vi "re_LuaVIEW Run Task.vi"(0 "script file or name (no name)":path, 5 "custom search directory (none)":path, 7 "script string (\"\" == load from file)":string, 9 "manual? (false)":bool, 11 "error in (no error)":errorcluster) -> (4 "manual error":bool, 8 "identifier":string, 15 "error out":errorcluster)   [LabVIEW 2012]
doc: "Runs a new LuaVIEW task. This prepares a task and runs it. This VI returns when the task has progressed beyond its initialization. When the task fails while initializing, its error is returned."
uses:
  typedefs/t_LuaVIEW Task State Instantiator Methods.ctl
  typedefs/t_LuaVIEW Task State Methods.ctl
  typedefs/t_LuaVIEW Task Modes.ctl
  typedefs/t_LuaVIEW Task Signals.ctl
  typedefs/t_LuaVIEW Prepared Script Infos Methods.ctl
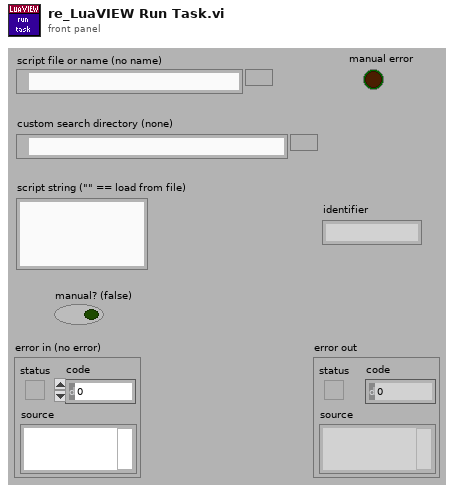
[diagram p1: front panel]
types:
  T1 = typedef "t_LuaVIEW Task State Instantiator Methods.ctl" = enum16{"instantiate", "isset", "retrieve"}
  T2 = typedef "t_LuaVIEW Task Modes.ctl" = enum16{"initializing", "running", "executing", "paused", "error", "swapping"}
  T3 = typedef "t_LuaVIEW Task State Methods.ctl" = enum16{"cleanup", "set initial", "set mode", "set active mode", "set error", "get task info", "get script info", "set signal", "clear signal", "test handled", "test delegated", "test signal", "handle signal", "delegate signal", "allow signal", "disallow signal", "disallow all", "signals?", "delegated signals?", "protection++", "protection--", "protection=0", "message", "next message", "pop message", "message available?", "force stop", "set swap preps", "apply swap preps"}
  T4 = typedef "t_LuaVIEW Task Signals.ctl" = enum32{"resume", "pause", "swap", "stop", "confirm"}
  T5 = typedef "t_LuaVIEW Prepared Script Infos Methods.ctl" = enum16{"isempty?", "empty", "set", "discard"}
  T6 = typedef "t_LuaVIEW Task State Pane.ctl" = refnum<vi>
  T7 = typedef "LuaVIEW Task Info.ctl" = cluster{"main script":string, "identifier":string, "class":string, "description":string, "mode":T2, "handler":string, "LuaVIEW reference":T8, "scripts":i32, "hide":bool, "active":bool, "error msg":string, "defer":bool, "launch":enum16{"asynchronous", "manual", "synchronous"}, "main path valid":bool, "start time":dbl, "swap time":dbl, "task VI":refnum<vi>, "prefsys":enum32{"invalid execution system", "user interface", "standard", "instrument i/o", "data acquisition", "other 1", "other 2", "same as caller"}, "priority":enum32{"invalid priority", "background priority", "normal priority", "above normal priority", "high priority", "time critical priority", "subroutine"}, "signal flags":u32, "allow mask":u32, "handle mask":u32, "disallow manual":bool}
  T8 = typedef "t_LuaVIEW Reference.ctl" = refnum<k1>
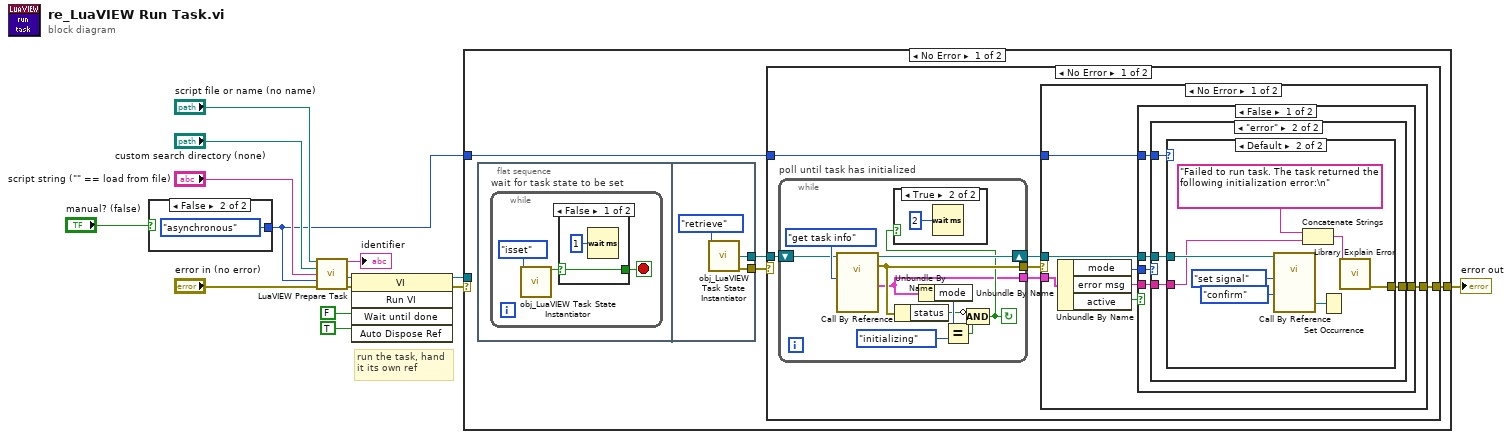
[diagram p0: block diagram]
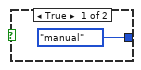
[diagram p2: hidden frame]
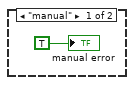
[diagram p6: hidden frame]
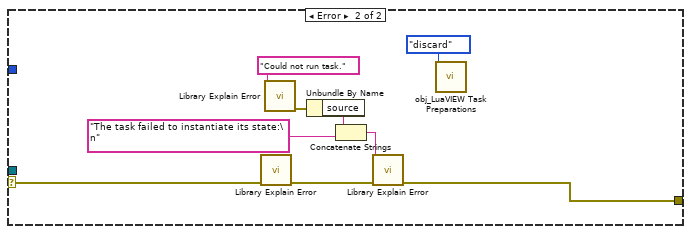
[diagram p9: hidden frame]
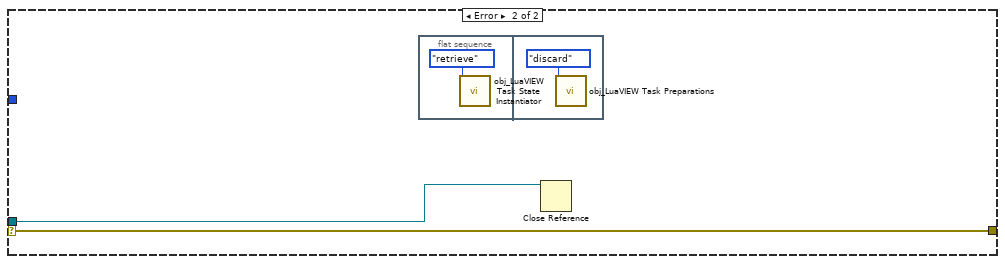
[diagram p10: hidden frame]
diagram:
  # "run the task, hand\nit its own ref"
  n1 = case shown="False" "manual? (false)" {
    tunnel: [enum16{"asynchronous", "manual", "synchronous"}."manual" ("launch mode") enum16{"asynchronous", "manual", "synchronous"}."asynchronous" ("launch mode")] -> w2
    frame True {
    }
    frame False {
    }
  }
  n2 = call "LuaVIEW Prepare Task.vi"("script file or name (no name)"="script file or name (no name)", "custom search directory (none)"="custom search directory (none)", "script string (\"\" == load from file)"="script string (\"\" == load from file)", "launch mode (whatever)"=w2, "error in (no error)"="error in (no error)") -> ("identifier"=→"identifier":string, "task instance"=w6:refnum<vi>, "error out"=w8:errorcluster)  [unwired: 8 in]
  n3 = invoke class="VI" method="Run VI"(reference=w6, error in=w8, "Wait until done"=FALSE, "Auto Dispose Ref"=TRUE) -> (reference out=w5:refnum<vi>, error out=w7:errorcluster)  [unwired: 1 in, 3 out]
  n4 = case shown="No Error" w7 {
    selector: w7 -> [_ w82]
    tunnel: [w20 w82] -> w14
    tunnel: w5 -> [_ w81]
    tunnel: w2 -> [w19 _]
    frame No Error {
      n5 = flat-sequence {
        tunnel: [w28] -> w18
        tunnel: [w27] -> w17
        frame #0 {
          n6 = while "wait for task state to be set" {
            stop <- w21 stop-if-true
            n7 = call "obj_LuaVIEW Task State Instantiator.vi"("method"=t_LuaVIEW_Task_State_Instantiator_Methods."isset") -> ("set for retrieval?"=w22:bool)  [unwired: 12 in, 2 out]
            n8 = case shown="False" w22 {
              selector: w22 -> [w24 w26]
              tunnel: [w24 w26] -> w21
              frame False {
                n9 = Wait (ms)(milliseconds to wait=u32 1) -> ()  [unwired: 1 out]
              }
              frame True {
              }
            }
          }
        }
        frame #1 {
          n10 = call "obj_LuaVIEW Task State Instantiator.vi"("method"=t_LuaVIEW_Task_State_Instantiator_Methods."retrieve") -> ("state object ref"=w27:T6, "instantiation error"=w28:errorcluster)  [unwired: 12 in, 1 out]
        }
      }
      n11 = case shown="No Error" w18 {
        selector: w18 -> [_ w79]
        tunnel: [w35 w72] -> w20
        tunnel: w19 -> [w31 _]
        tunnel: w17 -> [w30 _]
        frame No Error {
          n12 = while "poll until task has initialized" {
            shift-right: [w43] -> w32
            shift-left: w30 -> [w44]
            tunnel: [w38] -> w34
            tunnel: [w36] -> w33
            stop <- w37 continue-if-true
            n13 = call-by-ref "?"(reference=w44, "method"=t_LuaVIEW_Task_State_Methods."get task info") -> (reference out=w43:T6, error out=w38:errorcluster, "task info {get task info}"=w36:T7)  [unwired: 11 in, 4 out]
            n14 = Unbundle By Name(w38) -> ("status"=w40:bool)
            n15 = Unbundle By Name(w36) -> ("mode"=w41:T2)
            n16 = Equal?(x=w41, y=t_LuaVIEW_Task_Modes."initializing" ("mode")) -> (x = y?=w39:bool)
            n17 = Compound Arithmetic op=AND(invert w40, w39) -> (w37:bool)
            n18 = case shown="True" w37 {
              frame False {
              }
              frame True {
                n19 = Wait (ms)(milliseconds to wait=u32 2) -> ()  [unwired: 1 out]
              }
            }
          }
          n20 = case shown="No Error" w34 {
            tunnel: [w52 _] -> w35
            tunnel: w33 -> [w53 _]
            tunnel: w32 -> [w51 _]
            tunnel: w31 -> [w48 _]
            frame No Error {
              n21 = Unbundle By Name(w53) -> ("mode"=w49:T2, "error msg"=w50:string, "active"=w47:bool)
              n22 = case shown="False" w47 {
                tunnel: [w58 _] -> w52
                tunnel: w51 -> [w57 _]
                tunnel: w50 -> [w56 _]
                tunnel: w49 -> [w55 _]
                tunnel: w48 -> [w54 _]
                frame False {
                  n23 = case shown="\"error\"" w55 {
                    tunnel: [_ w61] -> w58
                    tunnel: w57 -> [_ w60]
                    tunnel: w56 -> [_ w62]
                    tunnel: w54 -> [_ w59]
                    frame Default {
                      # "Done initializing and no error yet.\nLeave the task to its own devices."
                    }
                    frame "error" {
                      n24 = case shown="Default" w59 {
                        tunnel: w62 -> [_ w64]
                        tunnel: [_ w71] -> w61
                        tunnel: w60 -> [_ w69]
                        frame "manual" {
                          "manual error" <- TRUE ("manual error")
                        }
                        frame Default {
                          n25 = call-by-ref "?"(reference=w69, "method"=t_LuaVIEW_Task_State_Methods."set signal", "signal"=t_LuaVIEW_Task_Signals."confirm") -> ("wakeup occurrence"=w66:refnum<k4>)  [unwired: 10 in, 6 out]
                          n26 = Concatenate Strings("Failed to run task. The task returned the following initialization error:\n" ("string"), w64) -> (w70:string)
                          n27 = Set Occurrence(w66) -> ()
                          n28 = call "Library Explain Error.vi"("explanation prefix (none)"=w70) -> ("explained error"=w71:errorcluster)  [unwired: 14 in]
                        }
                      }
                    }
                  }
                }
                frame True {
                  # "The task is active, errors will be\ndirected elsewhere."
                }
              }
            }
            frame Error {
              # "Task state reference no longer valid.\nThis means the task has cleaned up.\nThis is OK, it merely means that the\ntask was done rather quickly."
            }
          }
        }
        frame Error {
          n29 = call "Library Explain Error.vi"("error in (no error)"=w79) -> ("explained error"=w77:errorcluster)  [unwired: 14 in]
          n30 = call "Library Explain Error.vi"("explanation prefix (none)"="Could not run task.") -> ("explained error"=w76:errorcluster)  [unwired: 14 in]
          n31 = Unbundle By Name(w76) -> ("source"=w75:string)
          n32 = Concatenate Strings(w75, "The task failed to instantiate its state:\n" ("string")) -> (w73:string)
          n33 = call "Library Explain Error.vi"("explanation prefix (none)"=w73, "error in (no error)"=w77) -> ("explained error"=w72:errorcluster)  [unwired: 13 in]
          n34 = call "obj_LuaVIEW Task Preparations.vi"("method"=t_LuaVIEW_Prepared_Script_Infos_Methods."discard") -> ()  [unwired: 12 in, 3 out]
        }
      }
    }
    frame Error {
      n35 = flat-sequence {
        frame #0 {
          n36 = call "obj_LuaVIEW Task State Instantiator.vi"("method"=t_LuaVIEW_Task_State_Instantiator_Methods."retrieve") -> ()  [unwired: 12 in, 3 out]
        }
        frame #1 {
          n37 = call "obj_LuaVIEW Task Preparations.vi"("method"=t_LuaVIEW_Prepared_Script_Infos_Methods."discard") -> ()  [unwired: 12 in, 3 out]
        }
      }
      n38 = Close Reference(reference=w81) -> ()  [unwired: 1 in, 1 out]
    }
  }
  "error out" <- w14
